vi "example of p13-2.vi"() -> ()   [LabVIEW 2017]
panel:
  out "XY Graph":cluster{"Y":dbl[], "Y":dbl[]}[](graph)
  out "Array":i16[](array[numeric])
  out "number (0 to 1)":dbl
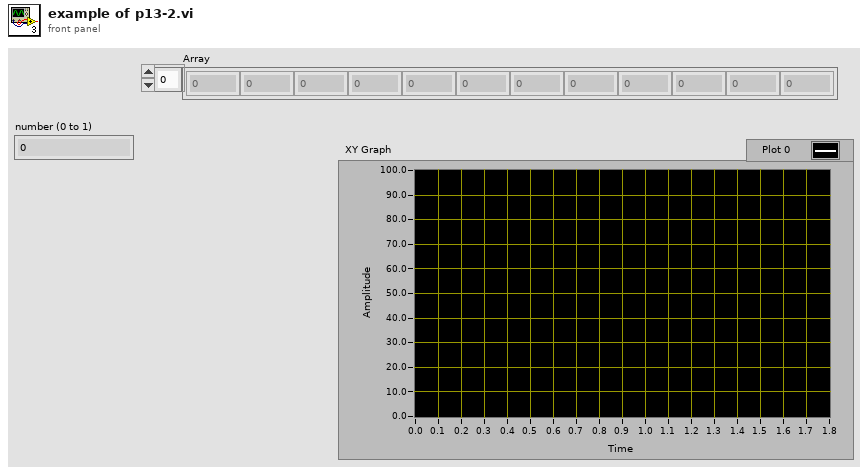
[diagram p1: front panel]
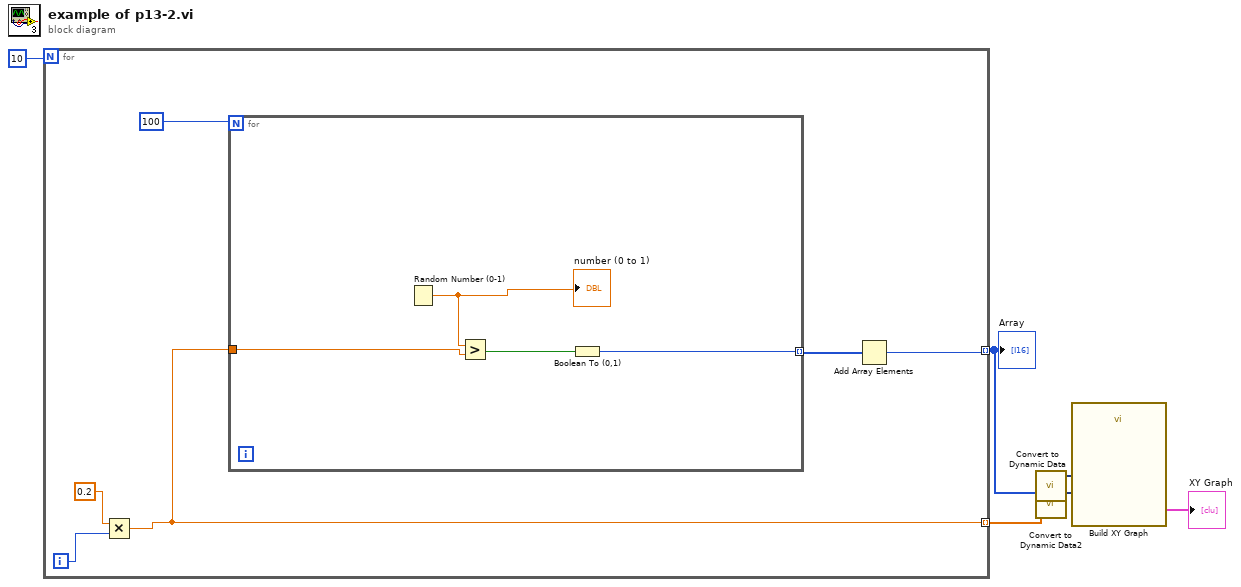
[diagram p0: block diagram]
diagram:
  n1 = for {
    N: 10 -> [_]
    tunnel: [w8] -> w2 mode=indexing
    tunnel: [w7] -> w4 mode=indexing
    i -> [w10]
    n2 = Multiply(x=0.2, y=w10) -> (x*y=w7:dbl)
    n3 = for {
      N: 100 -> [_]
      tunnel: [w14] -> w11 mode=indexing
      tunnel: w7 -> [w13]
      n4 = Random Number (0-1)() -> (number: 0 to 1=w16:dbl)
      "number (0 to 1)" <- w16
      n5 = Greater?(x=w16, y=w13) -> (0:w15:bool)
      n6 = Boolean To (0,1)(Boolean=w15) -> (0, 1=w14:i16)
    }
    n7 = Add Array Elements(numeric array=w11) -> (sum=w8:i16)
  }
  "Array" <- w2
  n8 = call "Convert to Dynamic Data"("Array"=w4) -> ("Dynamic Data Type"=w3:dynamicdata)  [unwired: 3 in]
  n9 = call "Convert to Dynamic Data2"("Array"=w2) -> ("Dynamic Data Type"=w1:dynamicdata)  [unwired: 3 in]
  n10 = call "Build XY Graph"("Y Input"=w1, "X Input"=w3) -> ("XY Graph"=→"XY Graph":cluster{"X":dbl[], "Y":dbl[]}[])  [unwired: 8 in, 1 out]
